vi "1021th frame-Set busy cursor.vi"(8 "error in (no error)":errorcluster, 9 "AVI mode":T1, 11 "Frame number":i32) -> (0 "error out":errorcluster, 2 "Busy cursor was set":bool)   [LabVIEW 2013]
uses:
  Typedefs/AVI implementation enum.ctl
  Globals/gl_Time series viewer globals.vi
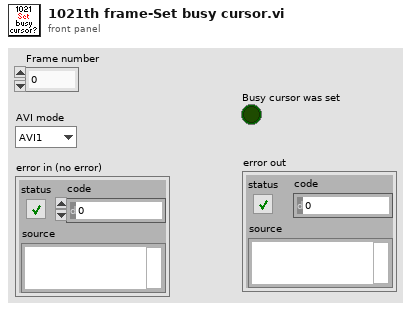
[diagram p1: front panel]
types:
  T1 = typedef "AVI implementation enum.ctl" = enum16{"AVI1", "AVI2"}
  T2 = typedef "Timelapse viewer refs.ctl" = cluster{"This VI":refnum<vi>, "AVI Mode ind":refnum<vi>, "Play":refnum<vi>, "Stop":refnum<vi>, "Back":refnum<vi>, "Scrollbar":refnum<vi>, "Video length info":refnum<vi>, "Expected speed values":refnum<vi>, "Intensity":refnum<vi>, "Path":refnum<vi>, "Selection sliders":refnum<vi>, "Speed Graph ref":refnum<vi>, "Frame rate set (fps)":refnum<vi>}
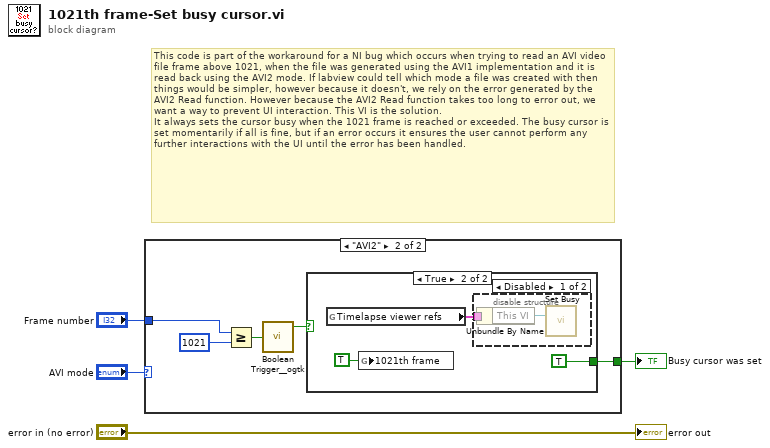
[diagram p0: block diagram]
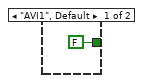
[diagram p2: hidden frame]
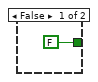
[diagram p3: hidden frame]
diagram:
  # "This code is part of the workaround for a NI bug which occurs when trying to read an AVI video file frame above 1021, when the file was generated using the AVI1 implementation and it is read back using the AVI2 mode. If labview could tell which mode a file was created with then things would be simpler, however because it doesn't, we rely on the error generated by the AVI2 Read function. However because the AVI2 Read function takes too long to error out, we want a way to prevent UI interaction. This VI is the solution.\nIt always sets the cursor busy when the 1021 frame is reached or exceeded. The busy cursor is set momentarily if all is fine, but if an error occurs it ensures the user cannot perform any further interactions with the UI until the error has been handled."
  n1 = case shown="\"AVI2\"" "AVI mode" {
    tunnel: "Frame number" -> [_ w8]
    tunnel: [FALSE w6] -> w1
    frame "AVI1", Default {
    }
    frame "AVI2" {
      n2 = Greater Or Equal?(x=w8, y=1021) -> (x >= y?=w9:bool)
      n3 = call "Boolean Trigger__ogtk.vi"("Boolean Input"=w9) -> ("Rising Edge"=w7:bool)  [unwired: 1 in, 1 out]
      n4 = case shown="True" w7 {
        tunnel: [FALSE TRUE] -> w6
        frame False {
        }
        frame True {
          n5 = global read "gl_Time series viewer globals.vi" "Timelapse viewer refs"() -> (w14:T2)
          n6 = global write "gl_Time series viewer globals.vi" "1021th frame"(TRUE ("1021th frame")) -> ()
          n7 = disable-structure shown="Disabled" {
            disable-tunnel: w14 -> [w16 _]
            frame Disabled {
              n8 = Unbundle By Name(w16) -> ("This VI"=w15:refnum<vi>)
              n9 = call <vilib>:"Set Busy.vi"("VI reference (current VI)"=w15) -> ()  [unwired: 9 in, 2 out]
            }
            frame Enabled {
            }
          }
        }
      }
    }
  }
  "Busy cursor was set" <- w1
  "error out" <- "error in (no error)"
